vi "ResetDSC.vi"(8 "error in (no error)":errorcluster, 11 "DSCNumber":u8) -> (0 "error out":errorcluster)   [LabVIEW 2015, in "ESLSCDLL.lvlib"]
uses:
  ESLSCDLL.lvlib
  Globals.vi
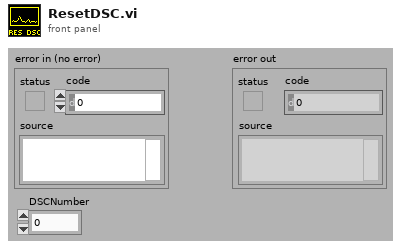
[diagram p1: front panel]
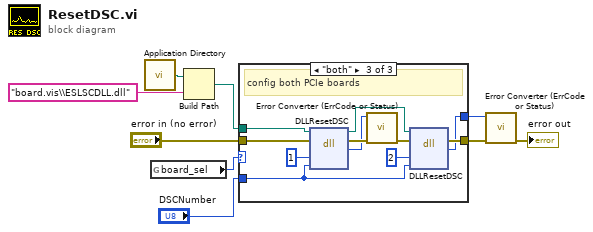
[diagram p0: block diagram]
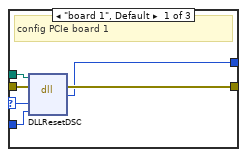
[diagram p2: hidden frame]
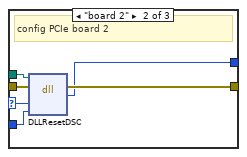
[diagram p3: hidden frame]
diagram:
  n1 = call <vilib>:"Application Directory.vi"() -> ("Application Directory"=w4:path)
  n2 = global read "Globals.vi" "board_sel"() -> (w5:enum32{"0", "board 1", "board 2", "both"})
  n3 = Build Path(base path=w4, name or relative path="board.vis\\ESLSCDLL.dll") -> (appended path=w2:path)
  n4 = case shown="\"both\"" w5 {
    selector: w5 -> [w15 w21 _]
    tunnel: "error in (no error)" -> [w14 w20 w30]
    tunnel: [w13 w19 w26] -> w7
    tunnel: [w12 w18 w25] -> w6
    tunnel: w2 -> [w11 w17 w24]
    tunnel: "DSCNumber" -> [w10 w16 w22]
    frame "board 1", Default {
      # "config PCIe board 1"
      n5 = dll-call lib="C:/ENTW/PCIE/LV64/board.vis/ESLSCDLL.dll" fn="DLLResetDSC" ("lwlscdll.dll:DLLWriteLongS0")(path in=w11, error in=w14, "drv"=w15, "DSCNumber"=w10) -> (error out=w13:errorcluster, "es_status_codes"=w12:i32)  [unwired: 3 in, 1 out]
    }
    frame "board 2" {
      # "config PCIe board 2"
      n6 = dll-call lib="C:/ENTW/PCIE/LV64/board.vis/ESLSCDLL.dll" fn="DLLResetDSC" ("lwlscdll.dll:DLLWriteLongS0")(path in=w17, error in=w20, "drv"=w21, "DSCNumber"=w16) -> (error out=w19:errorcluster, "es_status_codes"=w18:i32)  [unwired: 3 in, 1 out]
    }
    frame "both" {
      # "config both PCIe boards"
      n7 = dll-call lib="C:/ENTW/PCIE/LV64/board.vis/ESLSCDLL.dll" fn="DLLResetDSC" ("lwlscdll.dll:DLLWriteLongS0")(path in=w24, error in=w30, "drv"=u32 1, "DSCNumber"=w22) -> (path out=w23:path, error out=w29:errorcluster, "es_status_codes"=w28:i32)  [unwired: 3 in]
      n8 = call "Error Converter (ErrCode or Status).vi"("error in (no error)"=w29, "error code"=w28) -> ("error out"=w27:errorcluster)  [unwired: 9 in]
      n9 = dll-call lib="C:/ENTW/PCIE/LV64/board.vis/ESLSCDLL.dll" fn="DLLResetDSC" ("lwlscdll.dll:DLLWriteLongS0")(path in=w23, error in=w27, "drv"=u32 2, "DSCNumber"=w22) -> (error out=w26:errorcluster, "es_status_codes"=w25:i32)  [unwired: 3 in, 1 out]
    }
  }
  n10 = call "Error Converter (ErrCode or Status).vi"("error in (no error)"=w7, "error code"=w6) -> ("error out"=→"error out":errorcluster)  [unwired: 9 in]
